vi "labview3.vi"() -> ()   [LabVIEW 2019]
panel:
  in  "stop":bool
  out "return value":dbl[](array[numeric])
  out "Iteration counter":i32
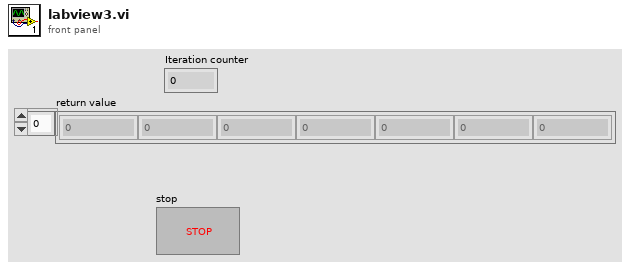
[diagram p1: front panel]
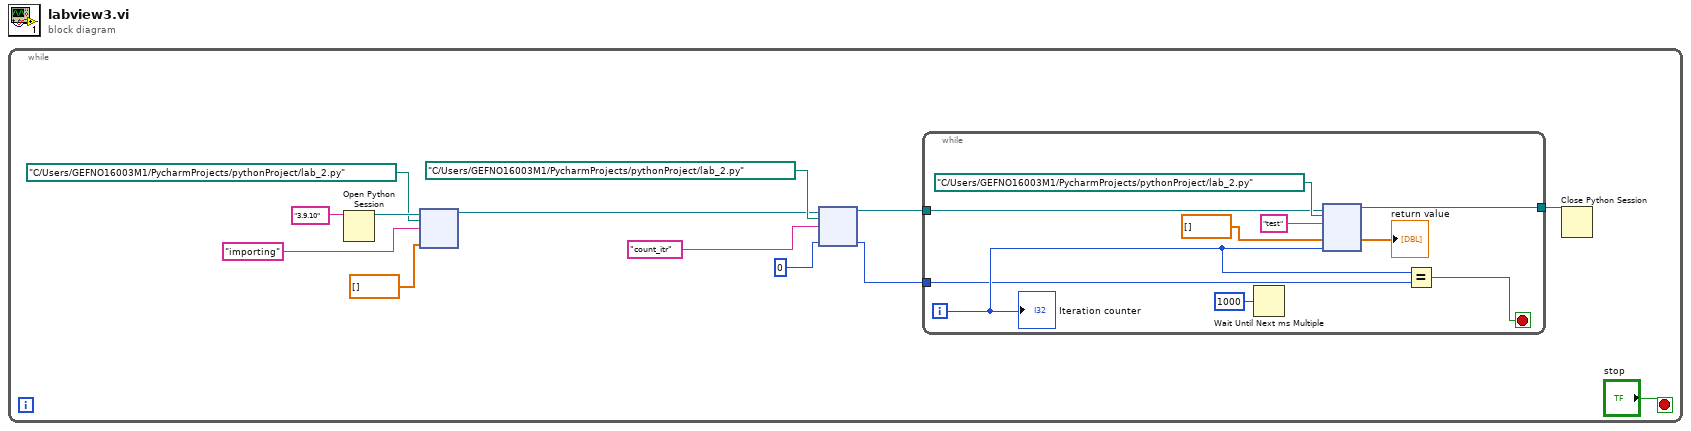
[diagram p0: block diagram]
diagram:
  n1 = while {
    stop <- "stop" stop-if-true
    n2 = Open Python Session(python version="3.9.10" ("Python version")) -> (session out=w13:refnum<k35>)  [unwired: 2 in, 1 out]
    n3 = node(w13, path "C:/Users/GEFNO16003M1/PycharmProjects/pythonProject/lab_2.py" ("module path"), "importing" ("function name"), dbl[] []) -> (w5:refnum<k35>)  [unwired: 2 in, 3 out]
    n4 = node(w5, path "C:/Users/GEFNO16003M1/PycharmProjects/pythonProject/lab_2.py" ("module path"), "count_itr" ("function name"), 0) -> (w4:refnum<k35>, w2:i32)  [unwired: 1 in, 3 out]
    n5 = while {
      tunnel: [w23] -> w9
      tunnel: w4 -> [w18]
      tunnel: w2 -> [w14]
      i -> [w20]
      stop <- w19 stop-if-true
      n6 = Wait Until Next ms Multiple(millisecond multiple=u32 1000) -> ()  [unwired: 1 out]
      n7 = node(w18, path "C:/Users/GEFNO16003M1/PycharmProjects/pythonProject/lab_2.py" ("module path"), "test" ("function name"), dbl[] [], w20) -> (w23:refnum<k35>, →"return value":dbl[])  [unwired: 2 in, 3 out]
      n8 = Equal?(x=w20, y=w14) -> (x = y?=w19:bool)
      "Iteration counter" <- w20
    }
    n9 = Close Python Session(session in=w9) -> ()  [unwired: 1 in, 1 out]
  }
